vi "Mass_2D_Plotter_MATLAB.vi"(1 "Job Directory":path=path "/G4_2_HD/Users/paulhayden/Documents/Projects/Hong Roughness/XW data/XW_Corr.tpt") -> (2 "Saved Automatically?":bool, 3 "Tex Info String":string, 4 "Plot data file":path)   [LabVIEW 2020]
uses:
  Results_plotter_Global.vi
  Globals/Constants_global.vi
  Data plotting/subVIs/Plot_Values_Global.vi
panel:
  out "Folder Paths":path[](array[path])
  out "Loop Number":i32
  out "Current Working on":string
  in  "stop":bool
  out "Folder Name":string
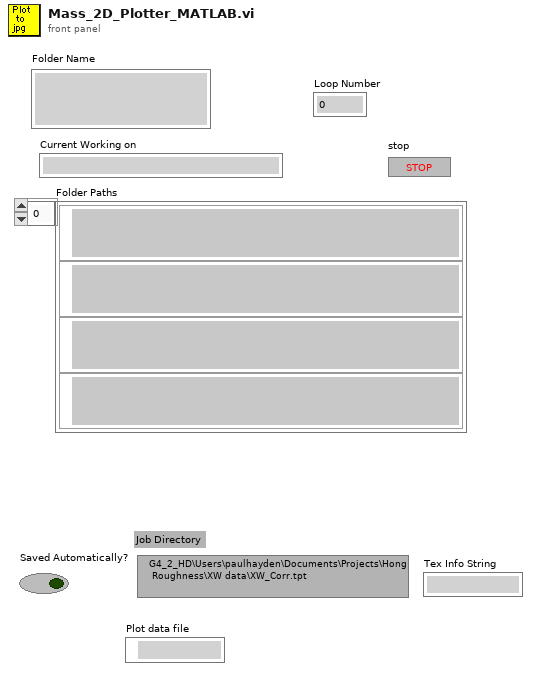
[diagram p1: front panel]
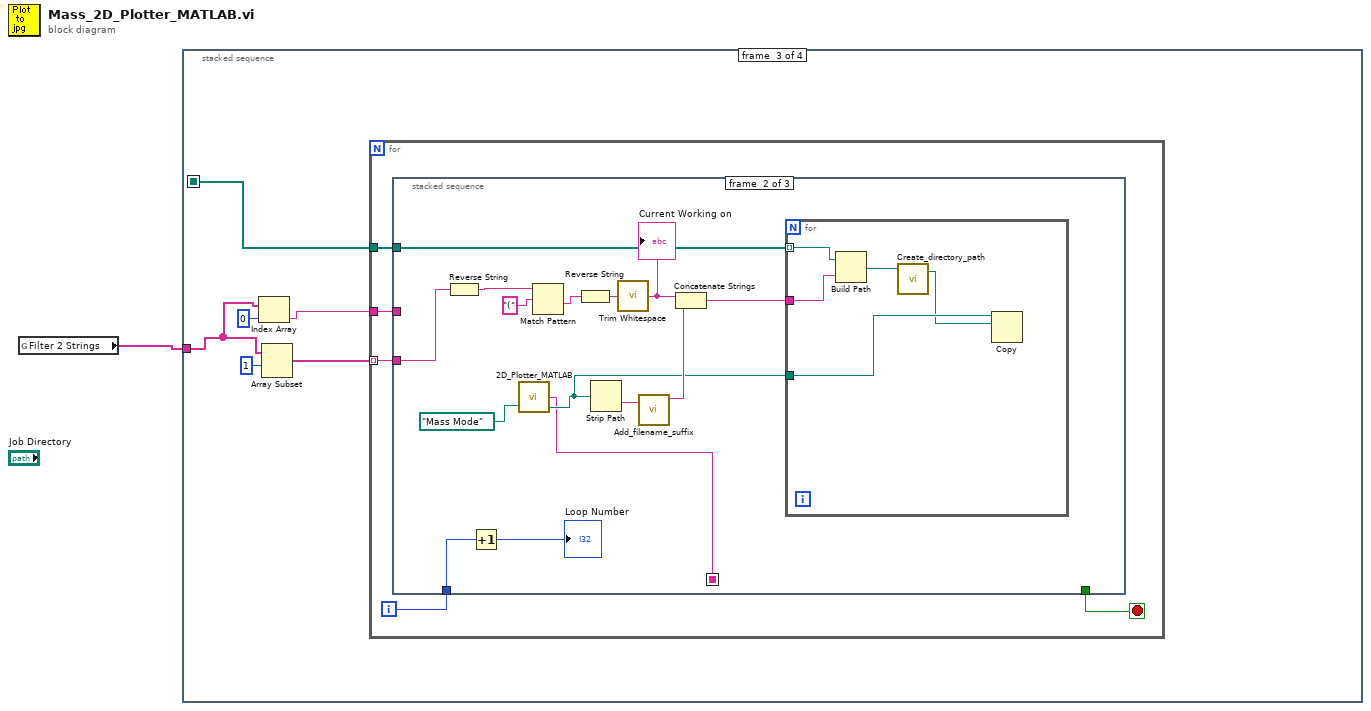
[diagram p0: block diagram]
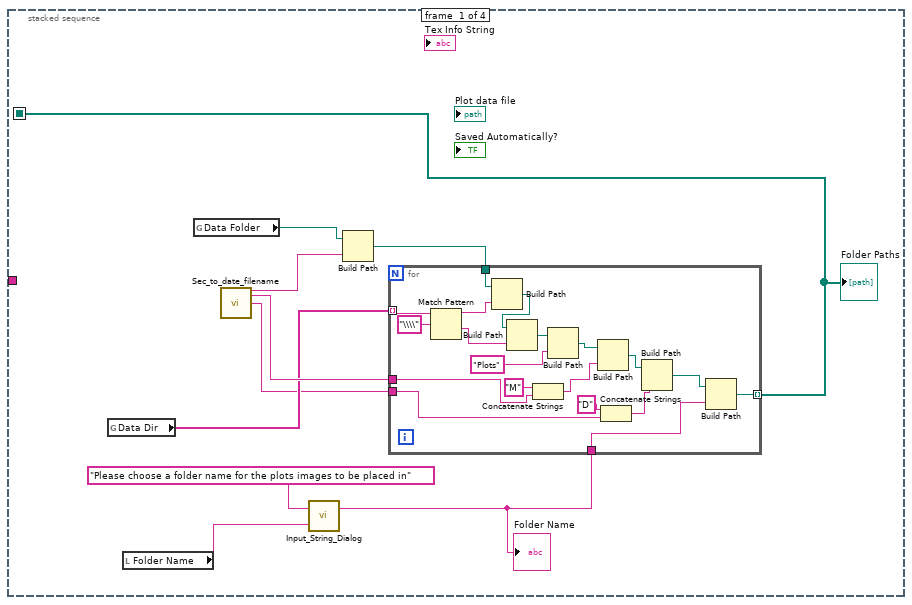
[diagram p2: hidden frame]
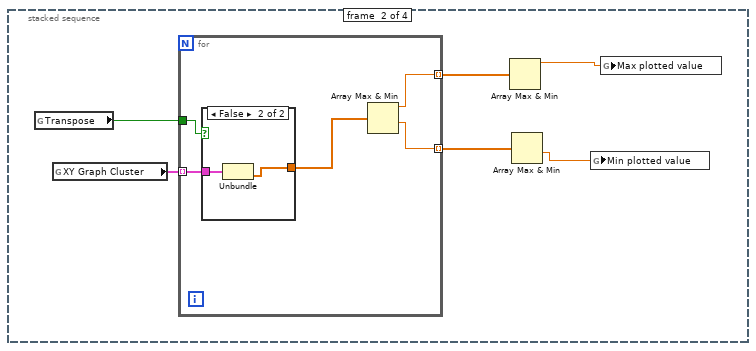
[diagram p3: hidden frame]
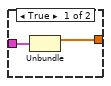
[diagram p4: hidden frame]
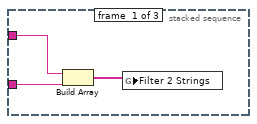
[diagram p5: hidden frame]
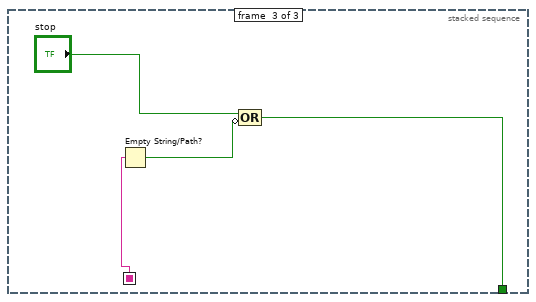
[diagram p6: hidden frame]
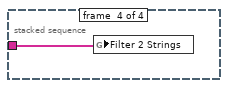
[diagram p7: hidden frame]
diagram:
  n1 = global read "Results_plotter_Global.vi" "Filter 2 Strings"() -> (w1:string[])
  n2 = stacked-sequence {
    seq-local: [w7 _ _ _] -> [_ _ w51 _]
    tunnel: w1 -> [_ _ w49 w84]
    frame #0 {
      n3 = global read "Results_plotter_Global.vi" "Data Dir"() -> (w6:string[])
      n4 = local read "Folder Name"() -> (w3:string)
      n5 = global read "Constants_global.vi" "Data Folder"() -> (w9:path)
      n6 = call "Sec_to_date_filename.vi"() -> ("HH:MM"=w11:string, "YYYY"=w8:string, "DD"=w2:string)  [unwired: 6 in, 7 out]
      n7 = call "Input_String_Dialog.vi"("Value"=w3, "Message to user"="Please choose a folder name for the plots images to be placed in") -> ("Output string"=w4:string)  [unwired: 1 out]
      "Folder Name" <- w4
      n8 = Build Path(base path=w9, name or relative path=w8) -> (appended path=w10:path)
      n9 = for {
        tunnel: w6 -> [w30] mode=indexing
        tunnel: w10 -> [w28]
        tunnel: w11 -> [w19]
        tunnel: w2 -> [w16]
        tunnel: w4 -> [w13]
        tunnel: [w12] -> w7 mode=indexing
        n10 = Match Pattern(string=w30, regular expression="\\\\") -> (before substring=w26:string, after substring=w25:string)  [unwired: 1 in, 2 out]
        n11 = Build Path(base path=w28, name or relative path=w26) -> (appended path=w27:path)
        n12 = Build Path(base path=w27, name or relative path=w25) -> (appended path=w24:path)
        n13 = Concatenate Strings("M" ("string"), w19) -> (w21:string)
        n14 = Build Path(base path=w24, name or relative path="Plots") -> (appended path=w22:path)
        n15 = Build Path(base path=w22, name or relative path=w21) -> (appended path=w18:path)
        n16 = Concatenate Strings("D" ("string"), w16) -> (w15:string)
        n17 = Build Path(base path=w18, name or relative path=w15) -> (appended path=w14:path)
        n18 = Build Path(base path=w14, name or relative path=w13) -> (appended path=w12:path)
      }
      "Folder Paths" <- w7
    }
    frame #1 {
      n19 = global read "Results_plotter_Global.vi" "Transpose"() -> (w31:bool)
      n20 = global read "Plot_Values_Global.vi" "XY Graph Cluster"() -> (w36:cluster{dbl[], dbl[]}[])
      n21 = for {
        tunnel: w36 -> [w41] mode=indexing
        tunnel: [w39] -> w35 mode=indexing
        tunnel: [w38] -> w34 mode=indexing
        tunnel: w31 -> [w37]
        n22 = case shown="False" w37 {
          tunnel: w41 -> [w43 w45]
          tunnel: [w42 w44] -> w40
          frame True {
            n23 = Unbundle(w43) -> (w42:dbl[])  [unwired: 1 out]
          }
          frame False {
            n24 = Unbundle(w45) -> (w44:dbl[])  [unwired: 1 out]
          }
        }
        n25 = Array Max & Min(array=w40) -> (max value=w39:dbl, min value=w38:dbl)  [unwired: 2 out]
      }
      n26 = Array Max & Min(array=w35) -> (max value=w33:dbl)  [unwired: 3 out]
      n27 = Array Max & Min(array=w34) -> (min value=w32:dbl)  [unwired: 3 out]
      n28 = global write "Results_plotter_Global.vi" "Min plotted value"(w32) -> ()
      n29 = global write "Results_plotter_Global.vi" "Max plotted value"(w33) -> ()
    }
    frame #2 {
      n30 = Index Array(array=w49, index=0) -> (element=w46:string)
      n31 = Array Subset(array=w49, index=1) -> (w47:string[])  [unwired: 1 in]
      n32 = for {
        tunnel: w51 -> [w56]
        tunnel: w47 -> [w55] mode=indexing
        tunnel: w46 -> [w54]
        i -> [w52]
        stop <- w53 stop-if-true
        n33 = stacked-sequence {
          seq-local: [_ w60 _] -> [_ _ w83]
          tunnel: w56 -> [_ w61 _]
          tunnel: w55 -> [w58 w65 _]
          tunnel: w54 -> [w57 _ _]
          tunnel: [_ _ w80] -> w53
          tunnel: w52 -> [_ w63 _]
          frame #0 {
            n34 = Build Array(w57, w58) -> (w59:string[])
            n35 = global write "Results_plotter_Global.vi" "Filter 2 Strings"(w59) -> ()
          }
          frame #1 {
            n36 = Reverse String(1:w65) -> (0:w69:string)
            n37 = Increment(x=w63) -> (x+1=→"Loop Number":i32)
            n38 = call "2D_Plotter_MATLAB.vi"("Job Directory"=path "Mass Mode") -> ("Error String"=w60:string, "Plot data file"=w70:path)  [unwired: 1 in, 1 out]
            n39 = Match Pattern(string=w69, regular expression="(") -> (after substring=w67:string)  [unwired: 1 in, 3 out]
            n40 = Reverse String(1:w67) -> (0:w66:string)
            n41 = Strip Path(path=w70) -> (name=w73:string)  [unwired: 1 out]
            n42 = call <vilib>:"Trim Whitespace.vi"("string"=w66) -> ("trimmed string"=w64:string)  [unwired: 1 in]
            "Current Working on" <- w64
            n43 = call "Add_filename_suffix.vi"("Filename"=w73) -> ("Original Suffix"=w72:string)  [unwired: 1 in, 3 out]
            n44 = Concatenate Strings(w64, w72) -> (w71:string)
            n45 = for {
              tunnel: w71 -> [w78]
              tunnel: w61 -> [w77] mode=indexing
              tunnel: w70 -> [w79]
              n46 = Build Path(base path=w77, name or relative path=w78) -> (appended path=w76:path)
              n47 = call "Create_directory_path.vi"("Path name"=w76) -> ("Path name Out"=w75:path)  [unwired: 2 in, 1 out]
              n48 = Copy(10:w75, 11:w79) -> ()  [unwired: 3 in, 3 out]
            }
          }
          frame #2 {
            n49 = Empty String/Path?(string/path=w83) -> (empty?=w81:bool)
            n50 = Compound Arithmetic op=OR("stop", invert w81) -> (w80:bool)
          }
        }
      }
    }
    frame #3 {
      n51 = global write "Results_plotter_Global.vi" "Filter 2 Strings"(w84) -> ()
    }
  }
